vi "Create.vi"(5 "Fake Project Inspector in":refnum<class "Fake Project Inspector.lvclass">, 8 "error in (no error)":errorcluster, 9 "Item Paths":path[](array[path]), 10 "Path":path, 11 "Name":string) -> (0 "error out":errorcluster, 3 "Fake Project Inspector":refnum<class "Fake Project Inspector.lvclass">)   [LabVIEW 2017, in "Cobertura.Tests.lvlib" / "Fake Project Inspector.lvclass"]
uses:
  Fake Project Inspector.lvclass
  Fake Project Inspector.lvclass/Fake Project Inspector.ctl
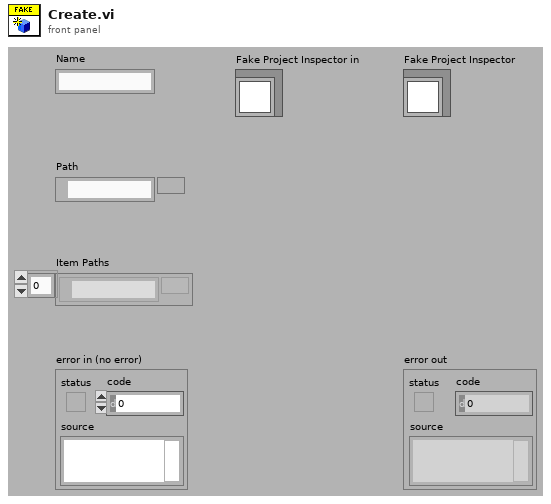
[diagram p1: front panel]
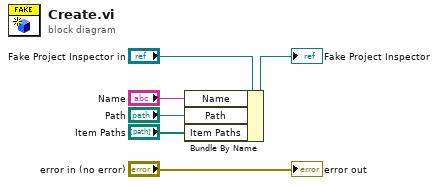
[diagram p0: block diagram]
diagram:
  n1 = Bundle By Name(cluster="Fake Project Inspector in", "Name"="Name", "Path"="Path", "Item Paths"="Item Paths") -> (→"Fake Project Inspector":refnum<class "Fake Project Inspector.lvclass">)
  "error out" <- "error in (no error)"
